vi "mlink_dio_set_func.vi"(8 "error in (no error)":errorcluster, 9 "state":T1, 10 "function":T2=enum."ENC1 (DIO1,DIO2)", 11 "connection ID":i32) -> (0 "error out":errorcluster, 3 "connection ID out":i32)   [LabVIEW 2009, in "MicroDAQ.lvlib" / "mlink.lvlib"]
doc: "This function controls DIO alternative functions. It enables or disables alternative DIO \nfunctions. By default all alternative DIO functions are enabled."
uses:
  <instrlib>/MicroDAQ/Mlink library wraper/mlink.lvlib
  <instrlib>/MicroDAQ/Tools/DIO Alternative functions.ctl
  <instrlib>/MicroDAQ/Tools/DIO set function argument.ctl
  <instrlib>/MicroDAQ/MLink32.dll
  <instrlib>/MicroDAQ/MicroDAQ.lvlib
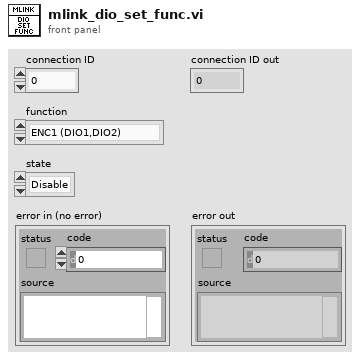
[diagram p1: front panel]
types:
  T1 = typedef "MicroDAQ.lvlib/DIO set function argument.ctl" = enum8{"Disable", "Enable"}
  T2 = typedef "MicroDAQ.lvlib/DIO Alternative functions.ctl" = enum8{"None", "ENC1 (DIO1,DIO2)", "ENC2 (DIO3, DIO4)", "PWM1 (DIO10, DIO11)", "PWM2 (DIO12, DIO13)", "PWM3 (DIO14, DIO15)", "UART (DIO8-Rx, DIO9-Tx)"}
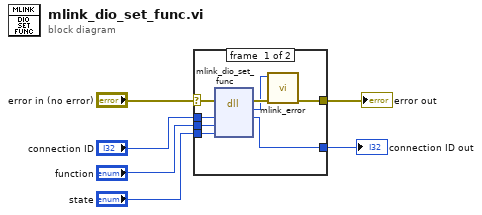
[diagram p0: block diagram]
diagram:
  n1 = case shown="No Error" "error in (no error)" {
    selector: "error in (no error)" -> [w12 w16]
    tunnel: "connection ID" -> [w14 w15]
    tunnel: [w13 w15] -> w5
    tunnel: "function" -> [w11 _]
    tunnel: "state" -> [w10 _]
    tunnel: [w7 w16] -> w3
    frame #0 {
      n2 = dll-call lib="C:/Program Files (x86)/National Instruments/LabVIEW 2009/instr.lib/MicroDAQ/MLink32.dll" fn="mlink_dio_set_func"(error in=w12, "connection ID"=w14, "function"=w11, "enable"=w10) -> (error out=w9:errorcluster, "return type"=w8:i32, "connection ID"=w13:i32)  [unwired: 4 in, 1 out]
      n3 = call <instrlib>:"mlink_error.vi"("error in (no error)"=w9, "error code"=w8) -> ("error out"=w7:errorcluster)  [unwired: 9 in]
    }
    frame #1 {
    }
  }
  "connection ID out" <- w5
  "error out" <- w3
